vi "Configure NI-SWITCH Custom Device.vi"() -> ()   [LabVIEW 2017]
uses:
  NI-SWITCH Examples.lvlib
  <vilib>/addons/VeriStand Custom Device Scripting APIs/NI-SWITCH/Scripting/NI-SWITCH Scripting.lvlib
  NationalInstruments.VeriStand.SystemDefinitionAPI
panel:
  in  "Topology":string(combo)="2510/Independent"
  in  "NI-SWITCH Module Name":string="PXI1Slot2"
  in  "Custom Device Name":string="NI-SWITCH"
  in  "Output System Definition file":path=path "System Definition Files/System Definition with NI-SWITCH.nivssdf"
  in  "Input System Definition File":path=path "System Definition Files/Default System Definition.nivssdf"
  # "Overview: Demonstrates using the NI-SWITCH custom device scripting API to configure an instance of the custom device. By default, the configuration is for an NI PXI-2510.\n\nInstructions:\n1. Browse to the system definition file to be used as input.\n2. Browse to a path to save the system definition file as output. This may be the same as the input file.\n3. Set the desired name of the custom device.\n4. Set the module name and the desired topology for the module.\n5. Run the VI and verify its results."
  # "System Definition Files"
  # "Custom Device Configuration"
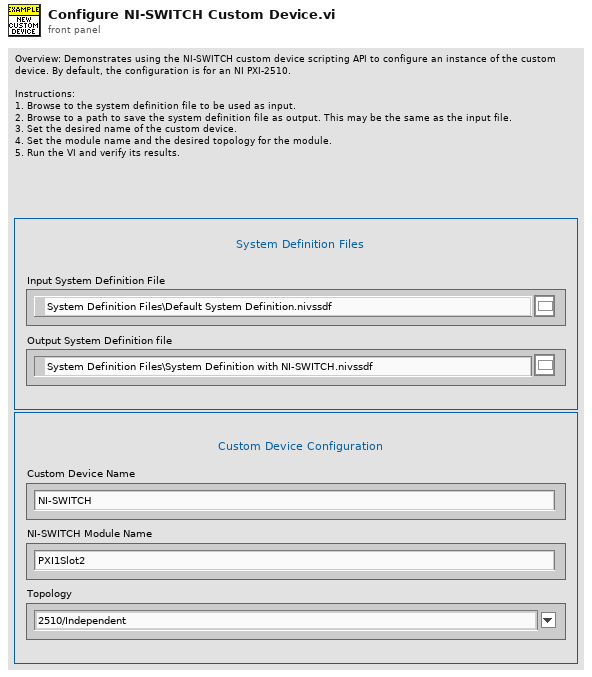
[diagram p1: front panel]
types:
  T1 = typedef "Custom Device API.lvlib/Custom Device Item Ref.ctl" = u64
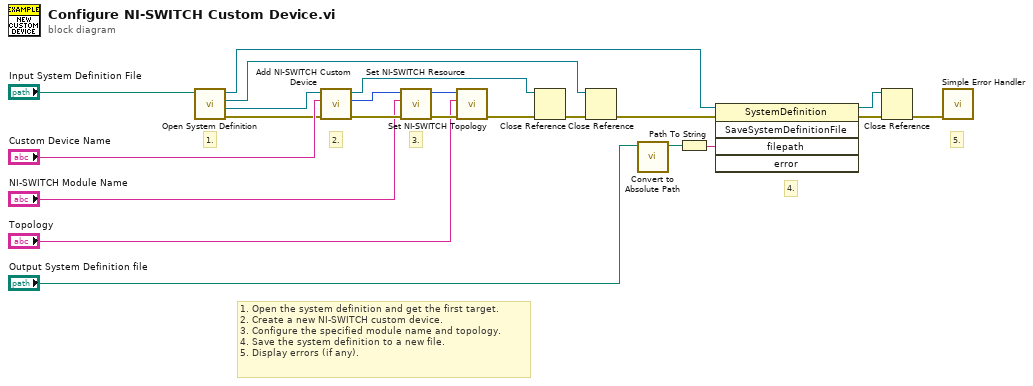
[diagram p0: block diagram]
diagram:
  # "3."
  # "2."
  # "1."
  # "4."
  # "5."
  # "1. Open the system definition and get the first target.\n2. Create a new NI-SWITCH custom device.\n3. Configure the specified module name and topology.\n4. Save the system definition to a new file.\n5. Display errors (if any)."
  n1 = call "Open System Definition.vi"("System Definition File"="Input System Definition File") -> ("error out"=w5:errorcluster, "Target Refnum"=w13:refnum<k24>, "Root Refnum"=w1:refnum<k24>, "System Definition Refnum"=w14:refnum<k24>)  [unwired: 7 in]
  n2 = call <vilib>:"Add NI-SWITCH Custom Device.vi"("error in"=w5, "name"="Custom Device Name", "target in"=w13) -> ("error out"=w12:errorcluster, "ni-switch custom device"=w10:T1, "target out"=w3:refnum<k24>)  [unwired: 6 in]
  n3 = call <vilib>:"Set NI-SWITCH Resource.vi"("error in"=w12, "resource"="NI-SWITCH Module Name", "ni-switch custom device in"=w10) -> ("error out"=w11:errorcluster, "ni-switch custom device out"=w9:T1)  [unwired: 7 in]
  n4 = call <vilib>:"Set NI-SWITCH Topology.vi"("error in"=w11, "topology"="Topology", "ni-switch custom device in"=w9) -> ("error out"=w18:errorcluster)  [unwired: 7 in, 1 out]
  n5 = Close Reference(reference=w3, error in (no error)=w18) -> (error out=w4:errorcluster)
  n6 = Close Reference(reference=w1, error in (no error)=w4) -> (error out=w2:errorcluster)
  n7 = call "Convert to Absolute Path.vi"("System Definition File"="Output System Definition file") -> ("Absolute Path"=w16:path)  [unwired: 10 in]
  n8 = Path To String(path=w16) -> (string=w22:string)
  n9 = invoke class="SystemDefinition" method="SaveSystemDefinitionFile"(reference=w14, error in=w2, "filepath"=w22) -> (reference out=w20:refnum<k24>, error out=w21:errorcluster)  [unwired: 2 in, 3 out]
  n10 = Close Reference(reference=w20, error in (no error)=w21) -> (error out=w17:errorcluster)
  n11 = call <vilib>:"Simple Error Handler.vi"("error in (no error)"=w17) -> ()  [unwired: 1 in, 8 out]
